vi "button position within vi.vi"(7 "VI with focus":refnum<vi>, 8 "error in (no error)":errorcluster, 10 "VI Reference":refnum<vi>, 11 "Boolean in":refnum<vi>) -> (0 "error out":errorcluster, 1 "Control found ?":bool, 2 "Vertical":i16, 3 "Horizontal":i16, 5 "Pane Refnum":refnum<vi>)   [LabVIEW 2020, in "ui-testing.lvlib"]
uses:
  ui-testing.lvlib
  <vilib>/Utility/miscctls.llb/LVPointTypeDef.ctl
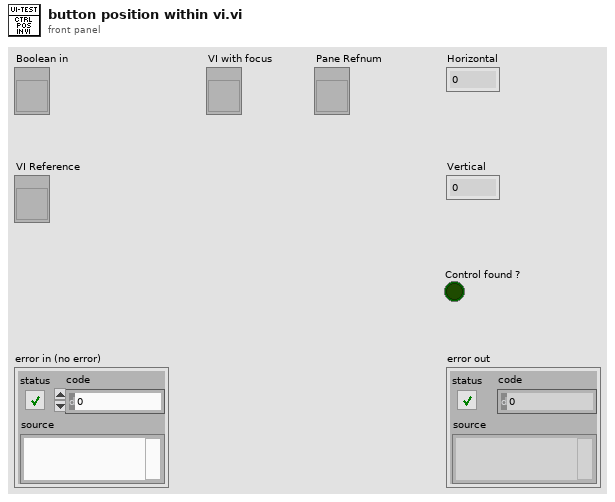
[diagram p1: front panel]
types:
  T1 = typedef "LVPointTypeDef.ctl" = cluster{"Horizontal":i16, "Vertical":i16}
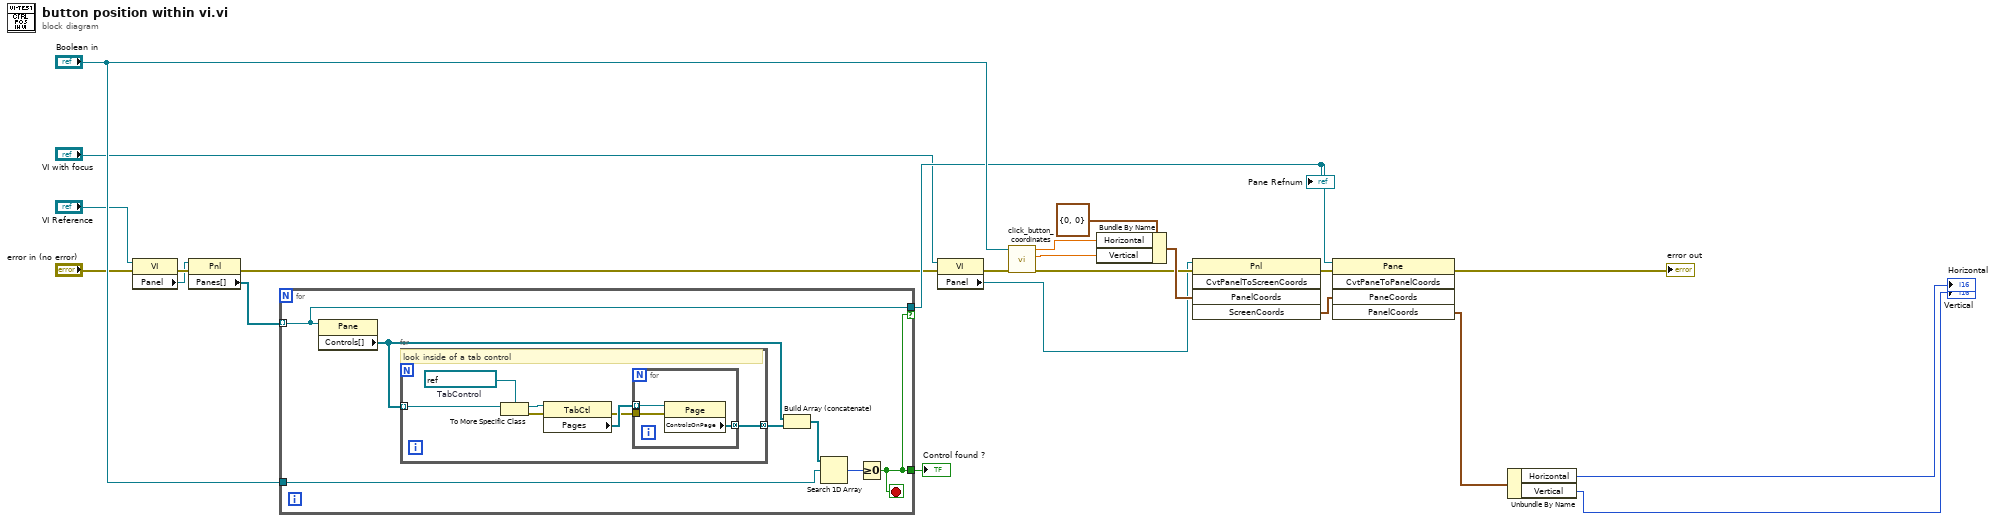
[diagram p0: block diagram]
diagram:
  n1 = property class="VI"(reference="VI Reference", error in="error in (no error)") -> (error out=w22:errorcluster, "Panel"=w11:refnum<vi>)  [unwired: 1 out]
  n2 = property class="Pnl"(reference=w11, error in=w22) -> (error out=w4:errorcluster, "Panes[]"=w23:refnum<vi>[])  [unwired: 1 out]
  n3 = for {
    tunnel: w23 -> [w29] mode=indexing
    tunnel: "Boolean in" -> [w30]
    tunnel: [w29] -> w16 if=w24
    tunnel: [w24] -> w5
    stop <- w24 stop-if-true
    n4 = property class="Pane"(reference=w29) -> ("Controls[]"=w26:refnum<vi>[])  [unwired: 1 in, 2 out]
    n5 = for {
      tunnel: w26 -> [w36] mode=indexing
      tunnel: [w31] -> w27 mode=concatenating
      w37 = refnum<vi> refnum  # TabControl
      # "look inside of a tab control"
      n6 = To More Specific Class(target class=w37, reference=w36) -> (specific class reference=w34:refnum<vi>, error out=w35:errorcluster)  [unwired: 1 in]
      n7 = property class="TabCtl"(reference=w34, error in=w35) -> (error out=w32:errorcluster, "Pages"=w33:refnum<vi>[])  [unwired: 1 out]
      n8 = for {
        tunnel: w33 -> [w40] mode=indexing
        tunnel: w32 -> [w39]
        tunnel: [w38] -> w31 mode=concatenating
        n9 = property class="Page"(reference=w40, error in=w39) -> ("ControlsOnPage"=w38:refnum<vi>[])  [unwired: 2 out]
      }
    }
    n10 = Build Array (concatenate)(w26, w27) -> (w25:refnum<vi>[])
    n11 = Search 1D Array(1D array=w25, element=w30) -> (index of element=w28:i32)  [unwired: 1 in]
    n12 = Greater Or Equal To 0?(x=w28) -> (x >= 0?=w24:bool)
  }
  "Control found ?" <- w5
  "Pane Refnum" <- w16
  n13 = property class="VI"(reference="VI with focus", error in=w4) -> (error out=w3:errorcluster, "Panel"=w2:refnum<vi>)  [unwired: 1 out]
  n14 = call "click_button_coordinates.vi"("error in (no error)"=w3, "Boolean in"="Boolean in") -> ("error out"=w10:errorcluster, "Vertical"=w15:dbl, "Horizontal"=w14:dbl)  [unwired: 7 in]
  n15 = Bundle By Name(cluster=T1 {"Horizontal"=0, "Vertical"=0} ("Panel Coordinates"), "Horizontal"=w14, "Vertical"=w15) -> (w13:T1)
  n16 = invoke class="Pnl" method="CvtPanelToScreenCoords"(reference=w2, error in=w10, "PanelCoords"=w13) -> (error out=w17:errorcluster, "ScreenCoords"=w18:T1)  [unwired: 2 in, 3 out]
  n17 = invoke class="Pane" method="CvtPaneToPanelCoords"(reference=w16, error in=w17, "PaneCoords"=w18) -> (error out=→"error out":errorcluster, "PanelCoords"=w20:T1)  [unwired: 2 in, 3 out]
  n18 = Unbundle By Name(w20) -> ("Horizontal"=→"Horizontal":i16, "Vertical"=→"Vertical":i16)
